vi "DSF.Shared.Configuration.Transfer Group.Get Direction.vi"(11 "Transfer Group Configuration in":refnum<class "DSF.Shared.Configuration.Transfer Group.lvclass">) -> (2 "direction":T1, 3 "Transfer Group Configuration out":refnum<class "DSF.Shared.Configuration.Transfer Group.lvclass">)   [LabVIEW 2017, in "DSF.Engine.lvlib" / "DSF.Shared.Configuration.Transfer Group.lvclass"]
uses:
  DSF.Shared.Configuration.Transfer Group.lvclass
  DSF Configuration API/1.0.0/Public/Controls/DSF Direction.ctl
  DSF.Shared.Configuration.Transfer Group.lvclass/DSF.Shared.Configuration.Transfer Group.ctl
  DSF Configuration API/1.0.0/DSF Configuration API.lvlib
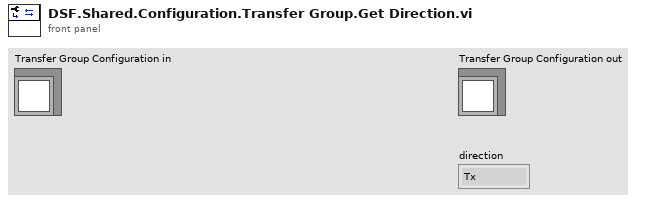
[diagram p1: front panel]
types:
  T1 = typedef "DSF Configuration API.lvlib/DSF Direction.ctl" = enum8{"Tx", "Rx"}
  T2 = typedef "DSF.Shared.Typedefs.Direction.ctl" = enum8{"Tx", "Rx"}
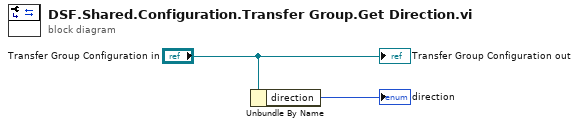
[diagram p0: block diagram]
diagram:
  n1 = Unbundle By Name("Transfer Group Configuration in") -> ("direction"=→"direction":T2)
  "Transfer Group Configuration out" <- "Transfer Group Configuration in"
